vi "X Position Image.vi"(8 "error in":errorcluster, 10 "Image In":T1) -> (0 "error out":errorcluster, 1 "Number of Matches (Shape Detection 1)":i32, 2 "Circles (Shape Detection 1)":T2(array[cluster]) {"Position"."Y" format="%.2f"; "Position"."X" format="%.2f"}, 3 "Image Out":T1)   [LabVIEW 2013]
uses:
  <vilib>/vision/Image Controls.llb/IMAQ Image.ctl
panel:
  # "Image in"
  # "Image out"
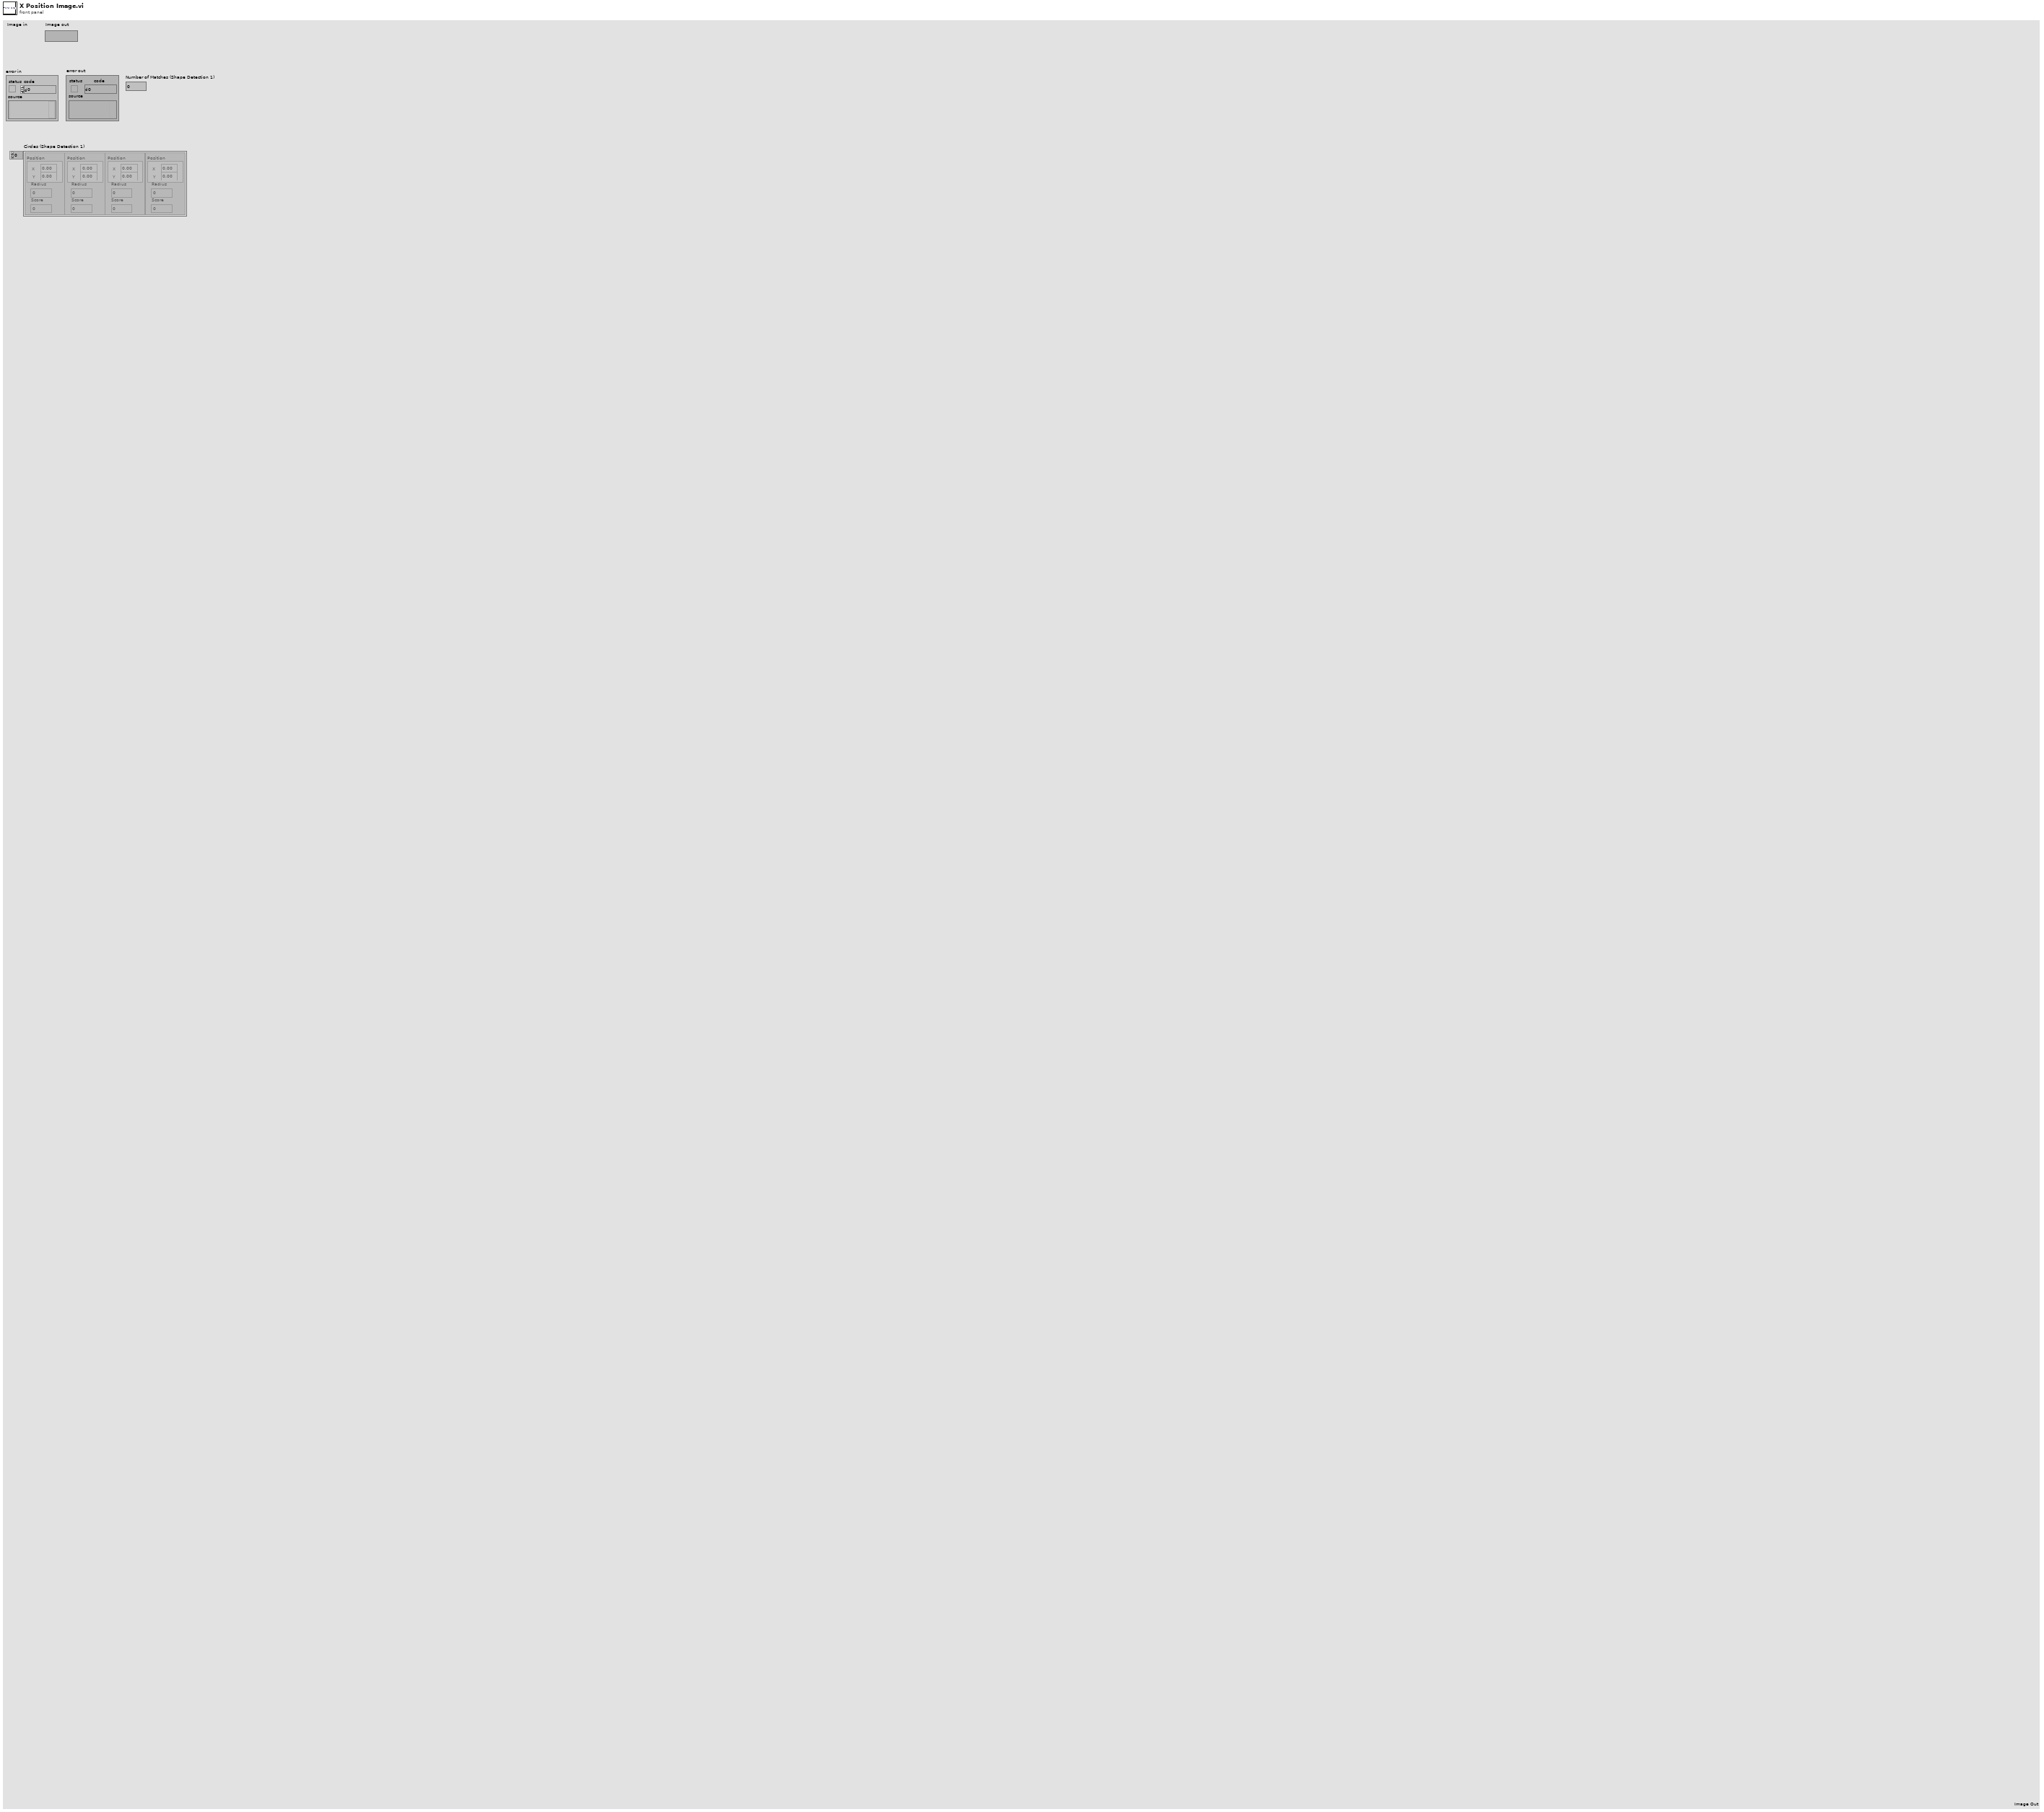
[diagram p1: front panel]
types:
  T1 = typedef "IMAQ Image.ctl" = refnum<image>
  T2 = cluster{"Position":cluster{"X":sgl, "Y":sgl}, "Radius":dbl, "Score":dbl}[]
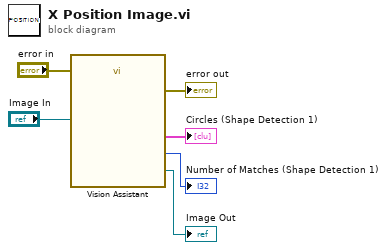
[diagram p0: block diagram]
diagram:
  n1 = call "Vision Assistant"("Image In"="Image In", "error in"="error in") -> ("Image Out"=→"Image Out":T1, "Circles (Shape Detection 1)"=→"Circles (Shape Detection 1)":T2, "Number of Matches (Shape Detection 1)"=→"Number of Matches (Shape Detection 1)":i32, "error out"=→"error out":errorcluster)  [unwired: 22 in]
